vi "PH_OceanOpticsSpectrometer.ProcEvents.vi"(0 "i ref in":refnum<vi>, 5 "error in":errorcluster) -> (14 "i ref out":refnum<vi>, 19 "error out":errorcluster)   [LabVIEW 2014, in "PH_OceanOpticsSpectrometer.lvlib"]
doc: "This method is used to define the events the object will listen to. Add your own events here."
uses:
  PH_OceanOpticsSpectrometer.lvlib
  CSCore/BaseProcess/BaseProcess.event definition.ctl
  CSCore/CAEObj/CAEObj.event definition.ctl
  CSCore/BaseProcess/BaseProcess.descriptor string definition.ctl
  CSCore/BaseProcess/BaseProcess.lvlib
  CSCore/CAEObj/CAEObj.lvlib
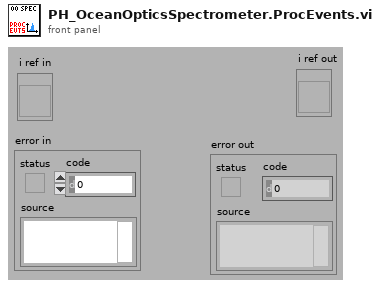
[diagram p1: front panel]
types:
  T1 = typedef "BaseProcess.lvlib/BaseProcess.event definition.ctl" = cluster{"CAEEvtDef":T2, "Data Descriptor":T3}
  T2 = typedef "CAEObj.lvlib/CAEObj.event definition.ctl" = cluster{"URL":string, "enable":bool, "ignoreResID":bool}
  T3 = typedef "BaseProcess.lvlib/BaseProcess.descriptor string definition.ctl" = string
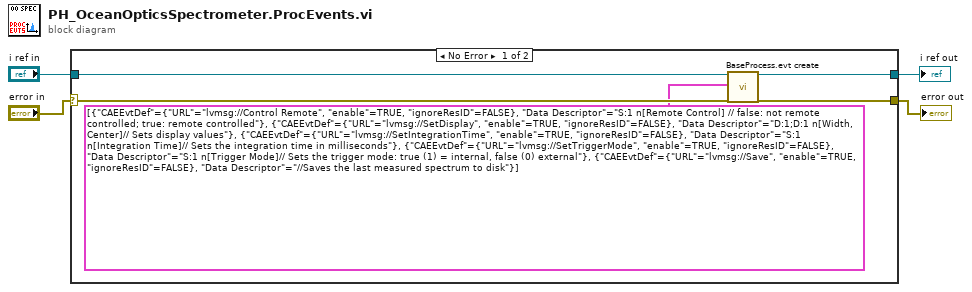
[diagram p0: block diagram]
diagram:
  n1 = case shown="No Error" "error in" {
    selector: "error in" -> [w6 w11]
    tunnel: [w9 w10] -> w4
    tunnel: [w8 w11] -> w3
    tunnel: "i ref in" -> [w7 w10]
    frame No Error {
      n2 = call "BaseProcess.evt create.vi"("i ref in"=w7, "newEvents"=T1[] [{"CAEEvtDef"={"URL"="lvmsg://Control Remote", "enable"=TRUE, "ignoreResID"=FALSE}, "Data Descriptor"="S:1 n[Remote Control] // false: not remote controlled; true: remote controlled"}, {"CAEEvtDef"={"URL"="lvmsg://SetDisplay", "enable"=TRUE, "ignoreResID"=FALSE}, "Data Descriptor"="D:1;D:1 n[Width, Center]// Sets display values"}, {"CAEEvtDef"={"URL"="lvmsg://SetIntegrationTime", "enable"=TRUE, "ignoreResID"=FALSE}, "Data Descriptor"="S:1 n[Integration Time]// Sets the integration time in milliseconds"}, {"CAEEvtDef"={"URL"="lvmsg://SetTriggerMode", "enable"=TRUE, "ignoreResID"=FALSE}, "Data Descriptor"="S:1 n[Trigger Mode]// Sets the trigger mode: true (1) = internal, false (0) external"}, {"CAEEvtDef"={"URL"="lvmsg://Save", "enable"=TRUE, "ignoreResID"=FALSE}, "Data Descriptor"="//Saves the last measured spectrum to disk"}] ("new events"), "error in (no error)"=w6) -> ("i ref out"=w9:refnum<vi>, "error out"=w8:errorcluster)  [unwired: 13 in, 2 out]
    }
    frame Error {
    }
  }
  "i ref out" <- w4
  "error out" <- w3
